vi "bank_account_withEvent.vi"() -> ()   [LabVIEW 2022 SP3]
panel:
  in  "Tab Control":enum32{"Page 1", "Page 2"}(tab)
  in  "Login Button":bool
  in  "Password":string
  in  "Username":string
  in  "ENTER":bool
  out "Balance":dbl
  in  "Menu":T1(ring)
  in  "Enter Money":dbl
  in  "Clear":bool
  in  "Logout":bool
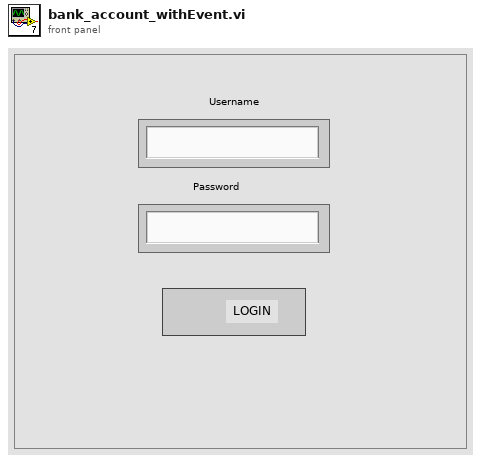
[diagram p1: front panel]
types:
  T1 = enum16{"", "Check Balance", "Cash Withdraw", "Cash Deposit"}
  T2 = enum8{"Enabled", "Disabled", "Disabled and Grayed Out"}
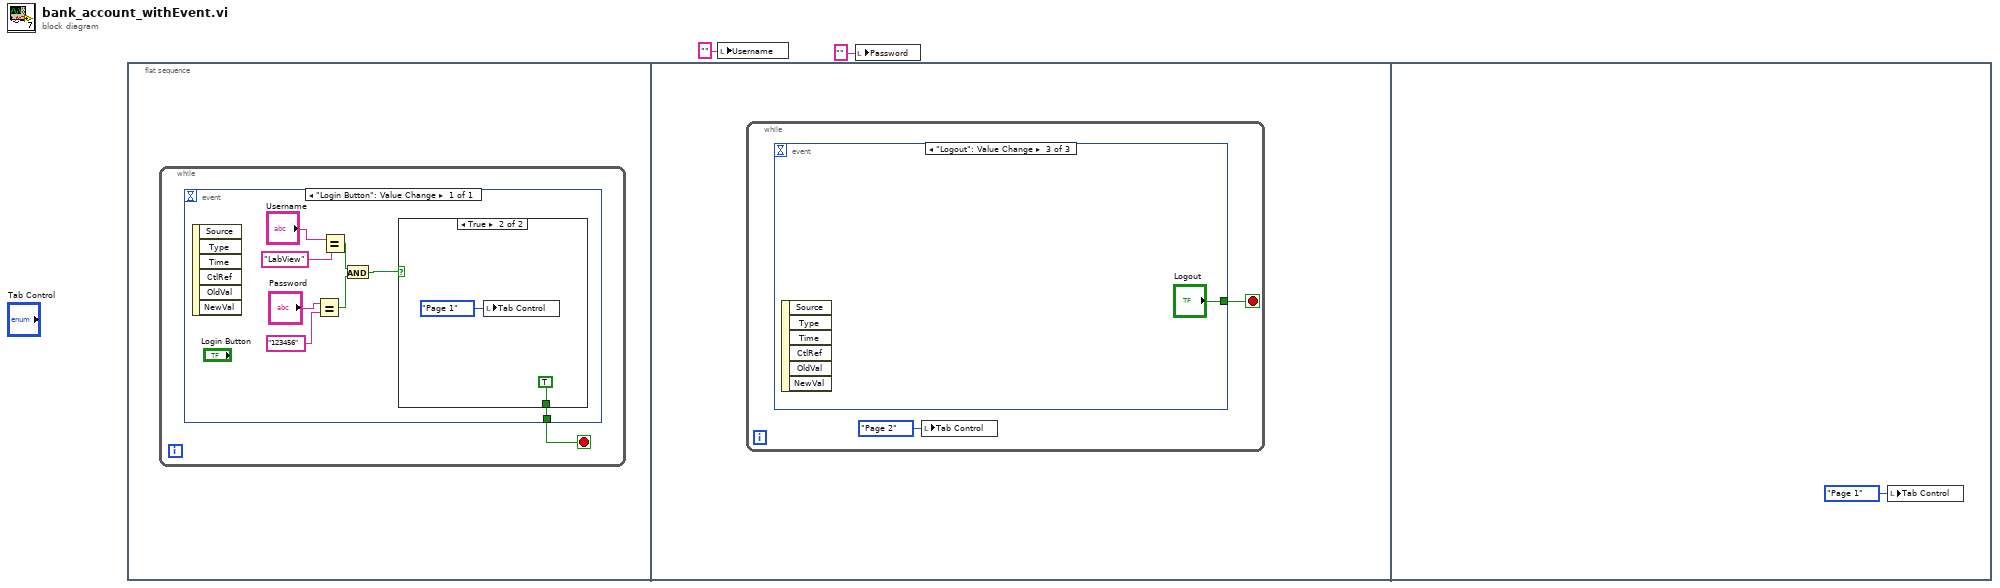
[diagram p0: block diagram]
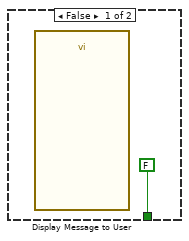
[diagram p2: hidden frame]
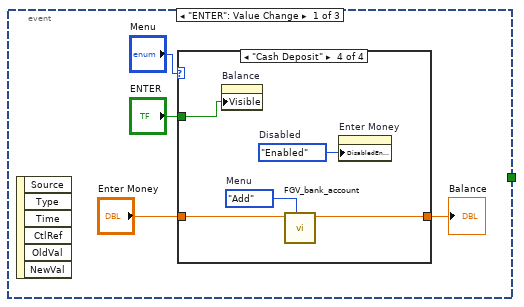
[diagram p3: hidden frame]
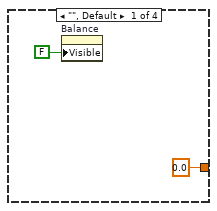
[diagram p4: hidden frame]
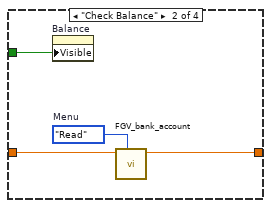
[diagram p5: hidden frame]
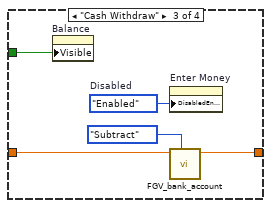
[diagram p6: hidden frame]
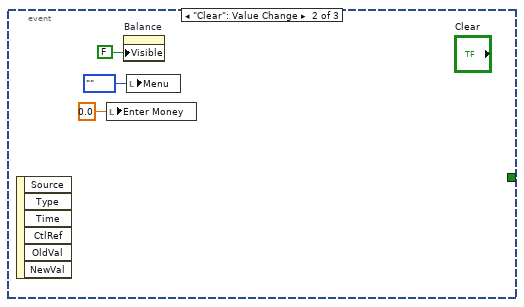
[diagram p7: hidden frame]
diagram:
  n1 = flat-sequence {
    frame #0 {
      n2 = while {
        stop <- w3 stop-if-true
        n3 = event shown="[0] \"Login Button\": Value Change" {
          selector: _ -> [_]
          dyn-events: _ -> [_]
          timeout: _ -> [_]
          tunnel: [w4] -> w3
          event "Login Button": Value Change {
            n4 = event-data() -> ()  [unwired: 1 in, 6 out]
            n5 = Equal?(x="Password", y="123456" ("x")) -> (x = y?=w5:bool)
            n6 = Equal?(x="Username", y="LabView") -> (x = y?=w6:bool)
            n7 = And(x=w6, y=w5) -> (x .and. y?=w7:bool)
            n8 = case shown="True" w7 {
              tunnel: [FALSE TRUE] -> w4
              frame False {
                n9 = call "Display Message to User"() -> ()  [unwired: 10 in, 2 out]
              }
              frame True {
                n10 = local write "Tab Control"(enum32{"Page 1", "Page 2"}."Page 1" ("Tab Control")) -> ()
              }
            }
          }
        }
      }
    }
    frame #1 {
      n11 = while {
        stop <- w15 stop-if-true
        n12 = event shown="[2] \"Logout\": Value Change" {
          selector: _ -> [_ _ _]
          dyn-events: _ -> [_ _ _]
          timeout: _ -> [_ _ _]
          tunnel: [_ _ "Logout"] -> w15
          event "ENTER": Value Change {
            n13 = event-data() -> ()  [unwired: 1 in, 6 out]
            n14 = case shown="\"Cash Deposit\"" "Menu" {
              tunnel: "Enter Money" -> [_ w25 w27 w34]
              tunnel: [0.0 w23 w28 w33] -> w18
              tunnel: "ENTER" -> [_ w26 w30 w35]
              frame "", Default {
                n15 = property on="Balance" class="DigNum (strict)"("Visible"=FALSE) -> ()  [unwired: 2 in, 2 out]
              }
              frame "Check Balance" {
                w24 = enum16{"Read", "Subtract", "Add"}."Read"  # Menu
                n16 = property on="Balance" class="DigNum (strict)"("Visible"=w26) -> ()  [unwired: 2 in, 2 out]
                n17 = call "FGV_bank_account.vi"("Menu"=w24, "input"=w25) -> ("Output"=w23:dbl)  [unwired: 8 in, 1 out]
              }
              frame "Cash Withdraw" {
                w31 = T2."Enabled"  # Disabled
                n18 = property on="Balance" class="DigNum (strict)"("Visible"=w30) -> ()  [unwired: 2 in, 2 out]
                n19 = property on="Enter Money" class="DigNum (strict)"("DisabledEnum"=w31) -> ()  [unwired: 2 in, 2 out]
                n20 = call "FGV_bank_account.vi"("Menu"=enum16{"Read", "Subtract", "Add"}."Subtract", "input"=w27) -> ("Output"=w28:dbl)  [unwired: 8 in, 1 out]
              }
              frame "Cash Deposit" {
                w32 = enum16{"Read", "Subtract", "Add"}."Add"  # Menu
                w36 = T2."Enabled"  # Disabled
                n21 = property on="Balance" class="DigNum (strict)"("Visible"=w35) -> ()  [unwired: 2 in, 2 out]
                n22 = call "FGV_bank_account.vi"("Menu"=w32, "input"=w34) -> ("Output"=w33:dbl)  [unwired: 8 in, 1 out]
                n23 = property on="Enter Money" class="DigNum (strict)"("DisabledEnum"=w36) -> ()  [unwired: 2 in, 2 out]
              }
            }
            "Balance" <- w18
          }
          event "Clear": Value Change {
            n24 = event-data() -> ()  [unwired: 1 in, 6 out]
            n25 = local write "Enter Money"(0.0 ("Enter Money")) -> ()
            n26 = property on="Balance" class="DigNum (strict)"("Visible"=FALSE) -> ()  [unwired: 2 in, 2 out]
            n27 = local write "Menu"(T1."" ("Menu")) -> ()
          }
          event "Logout": Value Change {
            n28 = event-data() -> ()  [unwired: 1 in, 6 out]
          }
        }
        n29 = local write "Tab Control"(enum32{"Page 1", "Page 2"}."Page 2" ("Tab Control")) -> ()
      }
    }
    frame #2 {
      n30 = local write "Tab Control"(enum32{"Page 1", "Page 2"}."Page 1" ("Tab Control")) -> ()
    }
  }
  n31 = local write "Username"("" ("Username")) -> ()
  n32 = local write "Password"("" ("Password")) -> ()
